vi "CommonVIs_UpdateMethodArguments.vi"(3 "CleanUpControls(True)":bool=TRUE, 4 "KeepLvClassInUpperRight/LeftCornerIfWired(True)":bool=TRUE, 5 "Always add ErrorIn/Out(True)":bool=TRUE, 6 "Keep Existing Controls And Indicatores connected(False)":bool, 7 "App":refnum<vi>, 8 "error in (no error)":errorcluster, 9 "MethodArguments":T1[](array[typedef]), 10 "ReturnType":T1, 11 "VI Ref/Vi Path":variant) -> (0 "error out":errorcluster)   [LabVIEW 2020]
uses:
  CommonVIs_AttributeType.ctl
  CommonVIs_AttributeDataType.ctl
  String/GDSString_AccessScopeModifierType.ctl
  SubVIs/GOOP_MethodArgumentType.ctl
  SubVIs/GOOP_MethodArgumentConnectionType.ctl
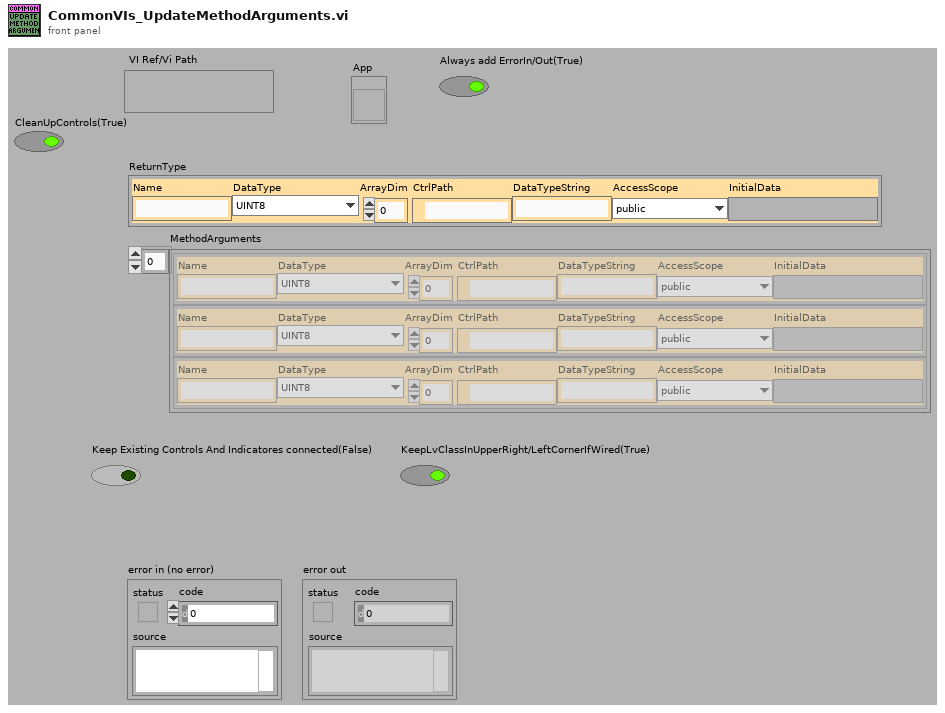
[diagram p1: front panel]
types:
  T1 = typedef "CommonVIs_AttributeType.ctl" = cluster{"Name":string, "DataType":T2, "ArrayDim":i32, "CtrlPath":path, "DataTypeString":string, "AccessScope":T3, "InitialData":variant}
  T2 = typedef "CommonVIs_AttributeDataType.ctl" = enum16{"UINT8", "INT8", "UINT16", "INT16", "UINT32", "INT32", "UINT64", "INT64", "SGL", "DBL", "EXT", "CSG", "CDB", "CXT", "TimeStamp", "STRING", "PATH", "BOOL", "ENUM", "RefNum", "VIRefNum", "LabVIEW Class", "Cluster", "Variant", "TypeDef", "Waveform", "LabVIEW Object", "Other", "void", "Set", "Map"}
  T3 = typedef "GDSString_AccessScopeModifierType.ctl" = enum16{"public", "private", "protected", "internal"}
  T4 = typedef "GOOP_MethodArgumentConnectionType.ctl" = enum16{"Required", "Recommended", "Optional", "Dynamic Dispatch"}
  T5 = typedef "GOOP_MethodArgumentType.ctl" = cluster{"Name":string, "DataType":T2, "ArrayDimensions":u8, "ConnectionType":T4, "DataTypeReference":path}
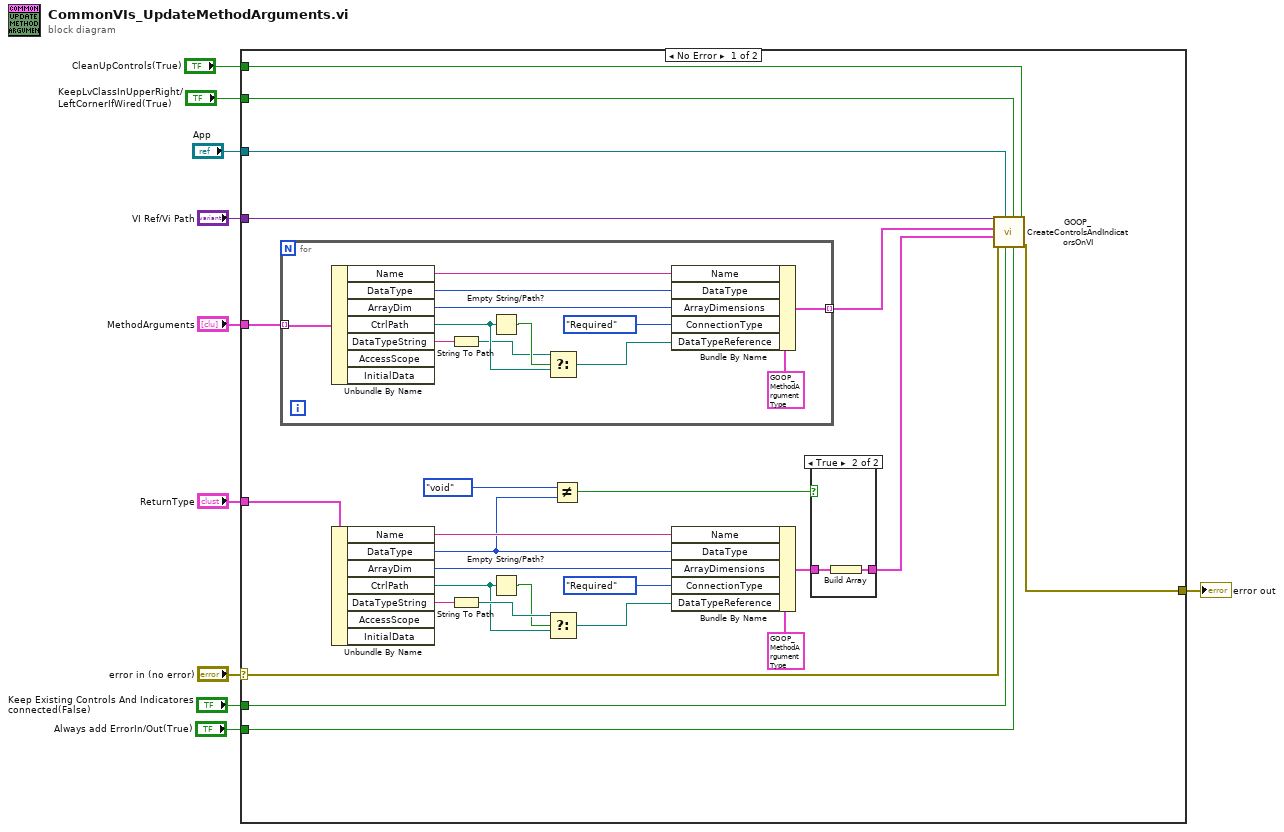
[diagram p0: block diagram]
diagram:
  n1 = case shown="No Error" "error in (no error)" {
    selector: "error in (no error)" -> [w34 w50]
    tunnel: [w19 w50] -> w9
    tunnel: "VI Ref/Vi Path" -> [w35 _]
    tunnel: "ReturnType" -> [w22 _]
    tunnel: "MethodArguments" -> [w33 _]
    tunnel: "App" -> [w18 _]
    tunnel: "Keep Existing Controls And Indicatores connected(False)" -> [w17 _]
    tunnel: "Always add ErrorIn/Out(True)" -> [w16 _]
    tunnel: "KeepLvClassInUpperRight/LeftCornerIfWired(True)" -> [w15 _]
    tunnel: "CleanUpControls(True)" -> [w11 _]
    frame No Error {
      n2 = for {
        tunnel: w33 -> [w49] mode=indexing
        tunnel: [w39] -> w32 mode=indexing
        n3 = Unbundle By Name(w49) -> ("Name"=w47:string, "DataType"=w38:T2, "ArrayDim"=w46:i32, "CtrlPath"=w42:path, "DataTypeString"=w44:string)  [unwired: 2 out]
        n4 = String To Path(string=w44) -> (path=w41:path)
        n5 = Empty String/Path?(string/path=w42) -> (empty?=w43:bool)
        n6 = Select(t=w41, s=w43, f=w42) -> (s? t:f=w40:path)
        n7 = Bundle By Name(cluster=T5 {"Name"="A", "DataType"=enum."UINT8", "ArrayDimensions"=1, "ConnectionType"=enum."Required", "DataTypeReference"=path ""} ("Argument"), "Name"=w47, "DataType"=w38, "ArrayDimensions"=w46, "ConnectionType"=GOOP_MethodArgumentConnectionType."Required", "DataTypeReference"=w40) -> (w39:T5)
      }
      n8 = Unbundle By Name(w22) -> ("Name"=w24:string, "DataType"=w13:T2, "ArrayDim"=w25:i32, "CtrlPath"=w29:path, "DataTypeString"=w27:string)  [unwired: 2 out]
      n9 = String To Path(string=w27) -> (path=w30:path)
      n10 = Empty String/Path?(string/path=w29) -> (empty?=w28:bool)
      n11 = Select(t=w30, s=w28, f=w29) -> (s? t:f=w31:path)
      n12 = Not Equal?(x=CommonVIs_AttributeDataType."void", y=w13) -> (x != y?=w12:bool)
      n13 = Bundle By Name(cluster=T5 {"Name"="A", "DataType"=enum."UINT8", "ArrayDimensions"=1, "ConnectionType"=enum."Required", "DataTypeReference"=path ""} ("Argument"), "Name"=w24, "DataType"=w13, "ArrayDimensions"=w25, "ConnectionType"=GOOP_MethodArgumentConnectionType."Required", "DataTypeReference"=w31) -> (w21:T5)
      n14 = case shown="True" w12 {
        tunnel: w21 -> [_ w37]
        tunnel: [_ w36] -> w20
        frame False {
        }
        frame True {
          n15 = Build Array(w37) -> (w36:T5[])
        }
      }
      n16 = call "GOOP_CreateControlsAndIndicatorsOnVI.vi"("CleanUpControls(True)"=w11, "Always add ErrorIn/Out(True)"=w16, "KeepLvClassInUpperRight/LeftCornerIfWired(True)"=w15, "Keep Existing Controls And Indicatores connected(False)"=w17, "App"=w18, "error in (no error)"=w34, "Indicators"=w20, "Controls"=w32, "VIRef/ViPath/ViName(in memory)"=w35) -> ("error out"=w19:errorcluster)  [unwired: 2 in]
    }
    frame Error {
    }
  }
  "error out" <- w9
